vi "main_EMD.vi"() -> ()   [LabVIEW 2018]
uses:
  <vilib>/Utility/file.llb/Read Delimited Spreadsheet (DBL).vi
  <vilib>/express/express analysis/Spectral/Block/exnSpectralBlock spectral measurements PSD poly.vi
  <vilib>/express/express analysis/Spectral/Block/exnSpectralBlock spectral measurements PSD WFM.vi
  <vilib>/express/express analysis/Spectral/XNode/ExpressSpectralMeasurementsBlockNode.xnode
  <vilib>/Analysis/NI_AALPro.lvlib
panel:
  out "PN50":dbl
  out "String":string
  out "LF/HF":dbl
  out "LF":dbl
  out "HF":dbl
  out "integral of P(x)":dbl
  out "Waveform Graph 3":cluster{"f0":dbl, "df":dbl, "magnitude":dbl[]}(graph)
  out "std(ms)":dbl[](array[numeric])
  out "R-R interval(ms)":dbl[](array[numeric])
  out "R wave time":dbl[](array[numeric])
  out "Heart Rate":dbl
  out "Waveform Graph 2":waveform(dbl)(graph)
  out "Ninth_IMF":dbl[](graph)
  out "Waveform Graph":dbl[][](graph)
  out "Eighth IMF":dbl[](graph)
  out "Seventh IMF":dbl[](graph)
  out "Sixth IMF":dbl[](graph)
  out "Fifth IMF":dbl[](graph)
  out "Num of IMF":i32
  out "original signal":dbl[](graph)
  in  "file path (dialog if empty)":path
  out "Fourth IMF":dbl[](graph)
  out "Third IMF":dbl[](graph)
  out "Second IMF":dbl[](graph)
  out "First IMF":dbl[](graph)
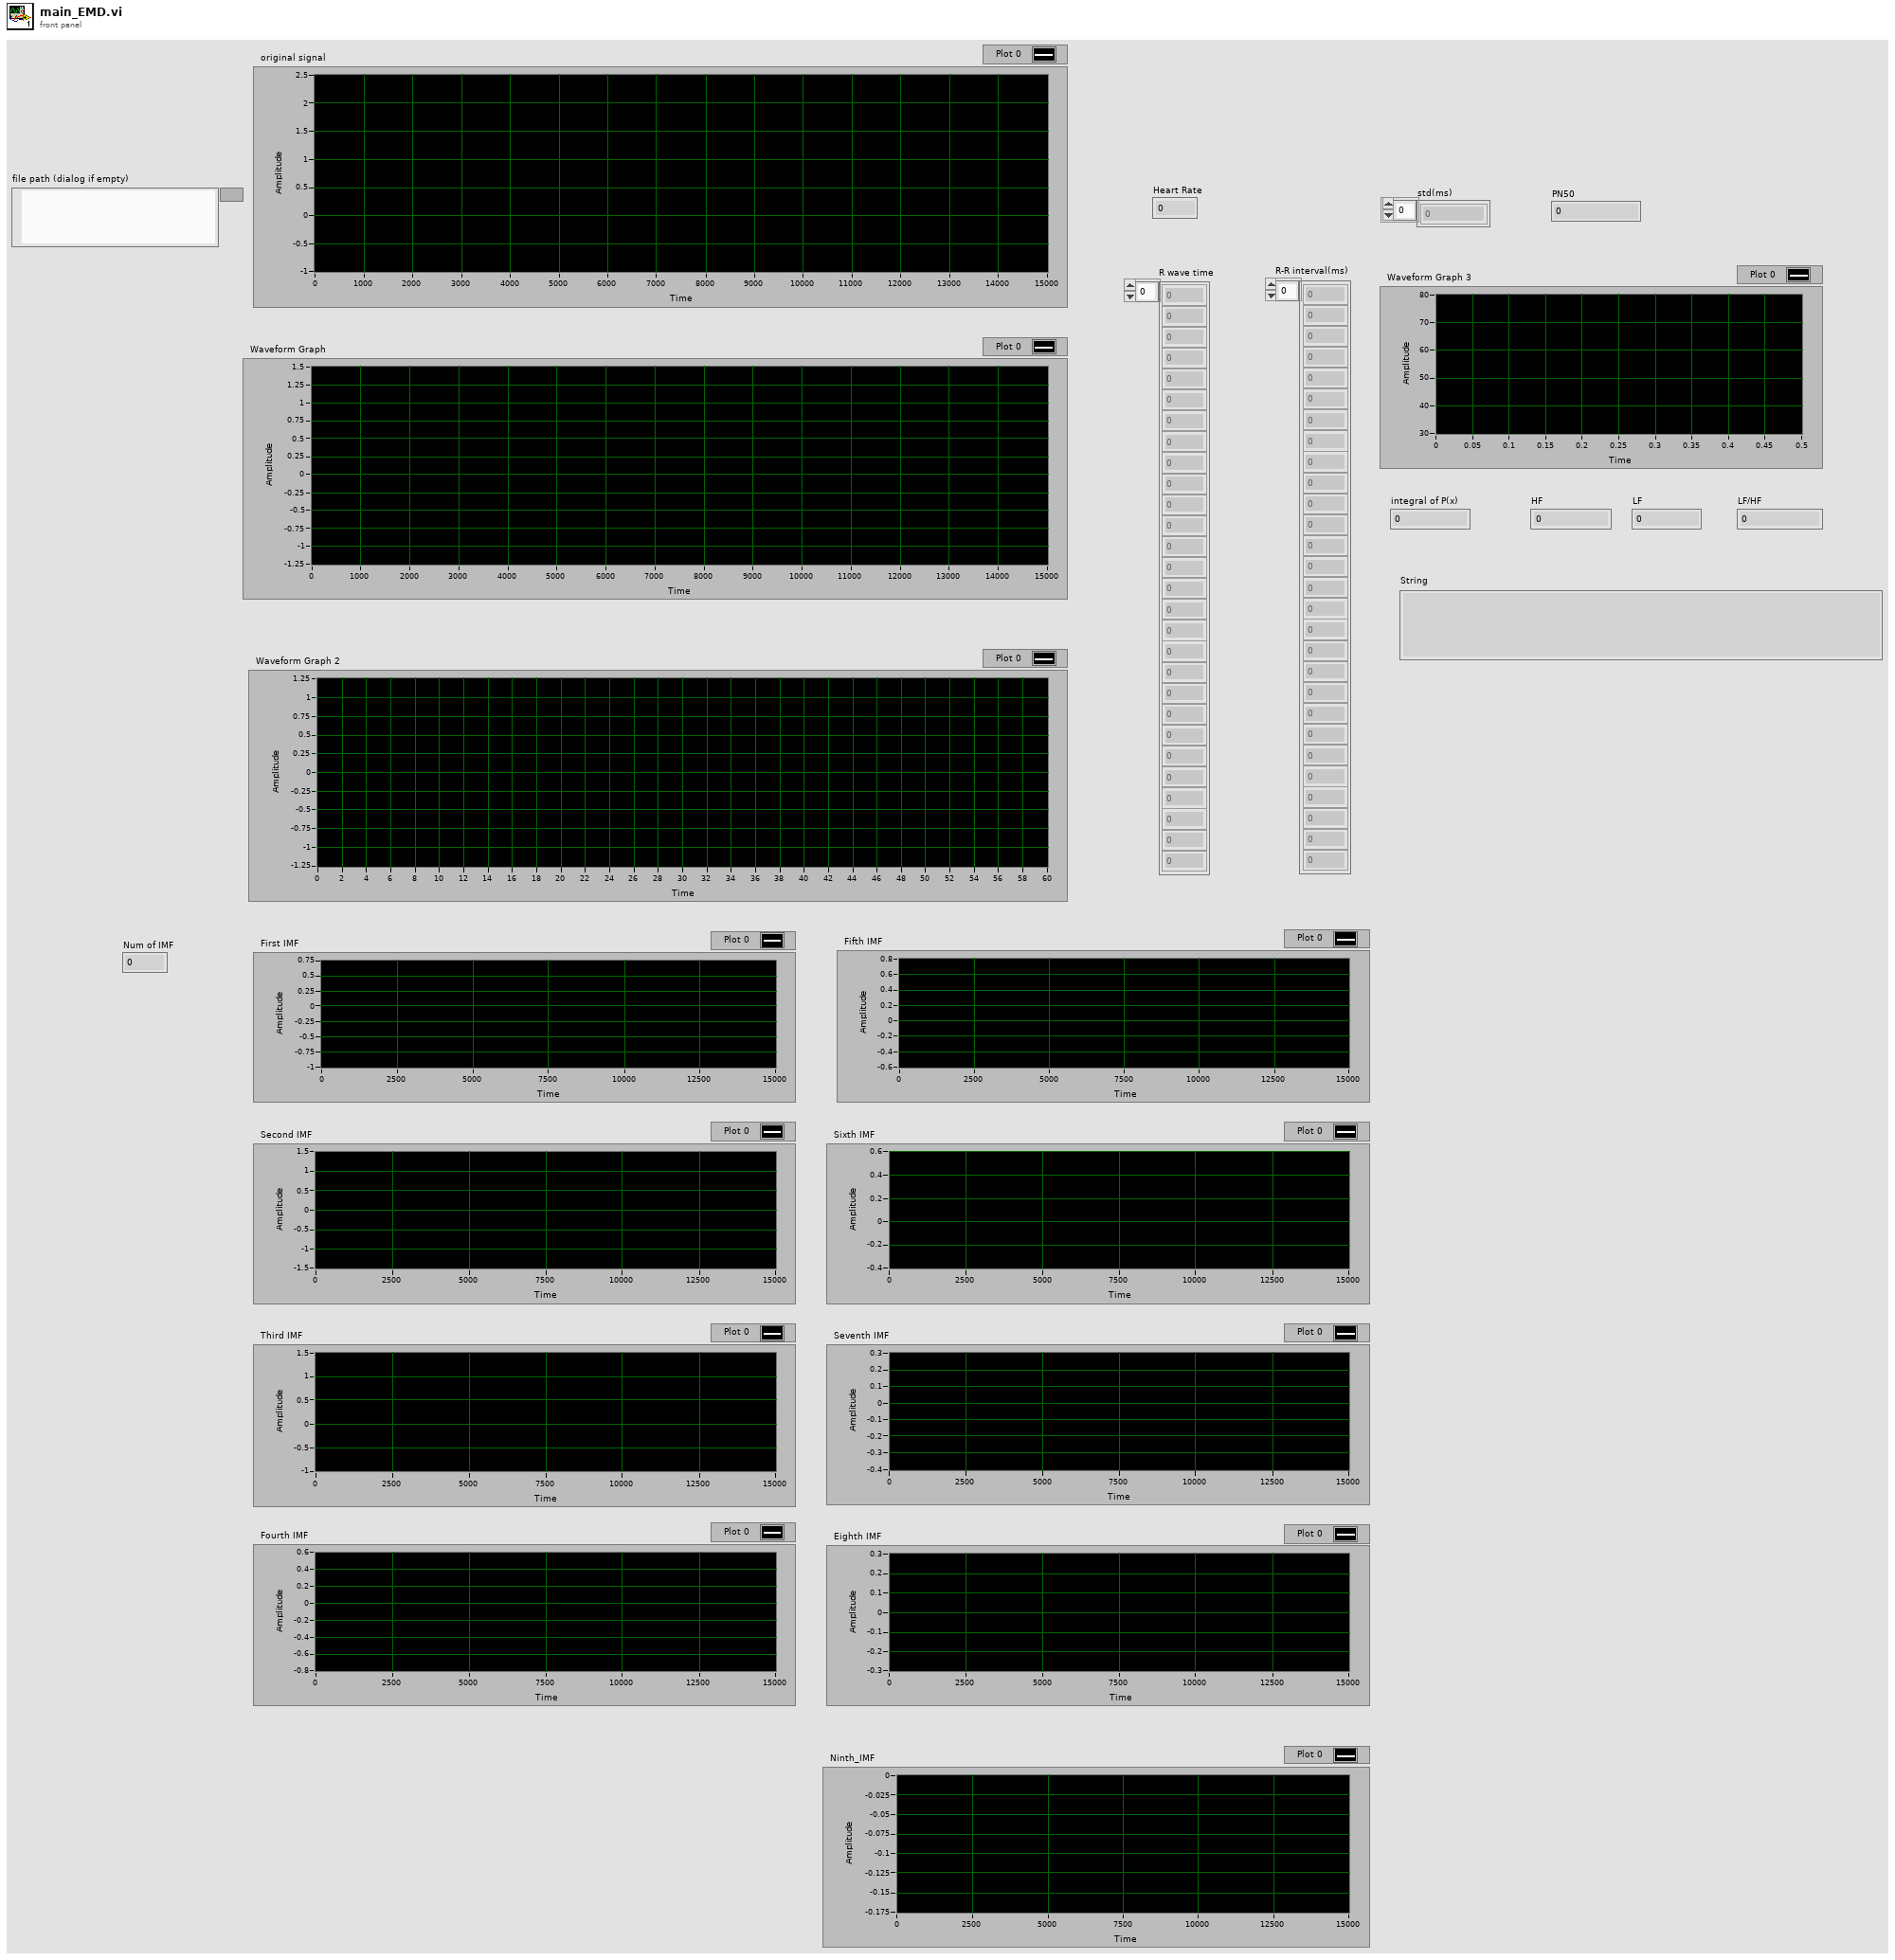
[diagram p1: front panel]
types:
  T1 = cluster{"averaging mode":u16, "weighting mode":u16, "number of averages":u32}
  T2 = cluster{"dB On (F)":bool, "unwrap phase (F)":bool, "convert to degree (F)":bool}
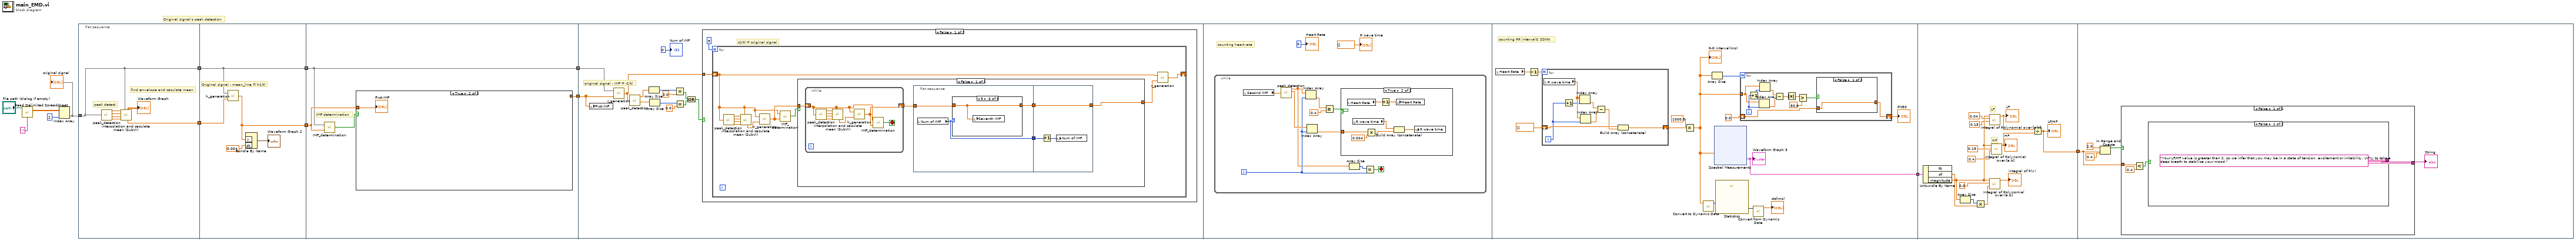
[diagram p0: block diagram]
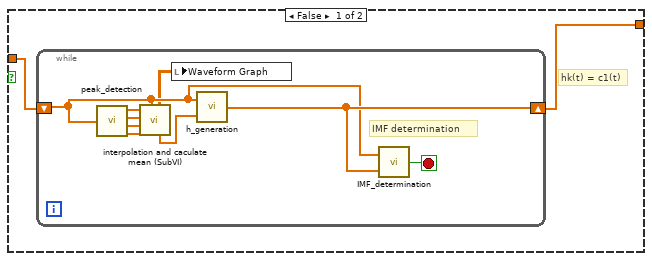
[diagram p2: hidden frame]
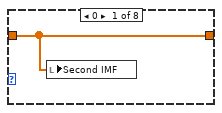
[diagram p3: hidden frame]
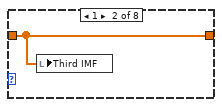
[diagram p4: hidden frame]
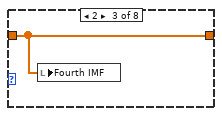
[diagram p5: hidden frame]
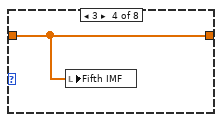
[diagram p6: hidden frame]
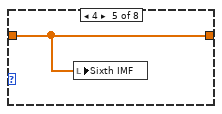
[diagram p7: hidden frame]
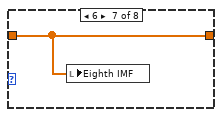
[diagram p8: hidden frame]
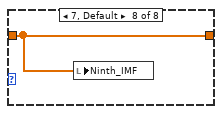
[diagram p9: hidden frame]
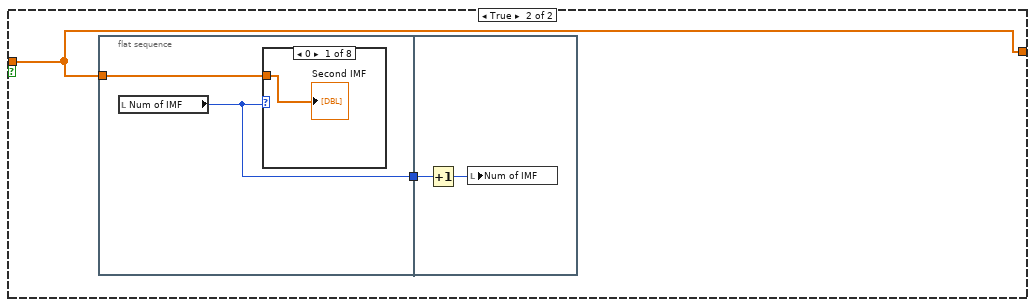
[diagram p10: hidden frame]
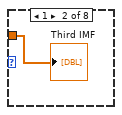
[diagram p11: hidden frame]
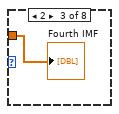
[diagram p12: hidden frame]
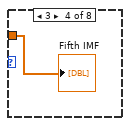
[diagram p13: hidden frame]
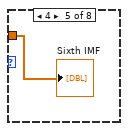
[diagram p14: hidden frame]
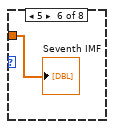
[diagram p15: hidden frame]
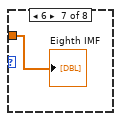
[diagram p16: hidden frame]
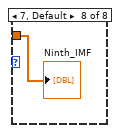
[diagram p17: hidden frame]
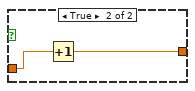
[diagram p20: hidden frame]
diagram:
  # "Original signal's peak detection"
  n1 = call-poly <vilib>:"Read Delimited Spreadsheet.vi"("file path (dialog if empty)"="file path (dialog if empty)", "delimiter (\\t)"=",") -> ("all rows"=w3:dbl[][])  [unwired: 8 in, 5 out]
  n2 = Index Array(array=w3, index (col)=2) -> (element=w4:dbl[])  [unwired: 1 in]
  "original signal" <- w4
  n3 = flat-sequence {
    tunnel: w4 -> [w20]
    tunnel: [w20] -> w13
    tunnel: [w15] -> w9
    tunnel: w13 -> [w25]
    tunnel: [w23] -> w12
    tunnel: [w25] -> w11
    tunnel: w9 -> [w24]
    tunnel: w12 -> [w28]
    tunnel: [w26] -> w8
    tunnel: w11 -> [w26]
    tunnel: [w29] -> w7
    tunnel: w8 -> [w44]
    tunnel: w7 -> [w43]
    tunnel: [w131] -> w2
    tunnel: w2 -> [w184]
    tunnel: [w171] -> w1
    tunnel: w1 -> [w185]
    frame #0 {
      # "peak detect"
      # "find envelope and caculate mean"
      n4 = call "peak_detection.vi"("Array"=w20) -> ("upper"=w19:dbl[], "upper time"=w18:dbl[], "lower"=w17:dbl[], "lower time"=w16:dbl[])
      n5 = call "interpolation and caculate mean (SubVI).vi"("upper"=w19, "upper time"=w18, "lower"=w17, "lower time"=w16, "original"=w20) -> ("up+mean+low"=→"Waveform Graph":dbl[][], "mean after interpolation"=w15:dbl[])  [unwired: 4 out]
    }
    frame #1 {
      # "Original signal - mean_line = h1(t)"
      n6 = call "h_generation.vi"("every_mean_points"=w24, "Y"=w25) -> ("h(t)"=w23:dbl[])
      n7 = Bundle By Name("Y"=w23, "dt"=0.004) -> (→"Waveform Graph 2":waveform(dbl))  [unwired: 1 in]
    }
    frame #2 {
      # "IMF determination"
      n8 = call "IMF_determination.vi"("h(t)"=w28, "original signal"=w26) -> ("x .and. y?"=w27:bool)
      n9 = case shown="True" w27 {
        tunnel: w28 -> [w31 w41]
        tunnel: [w30 _] -> w29
        frame False {
          # "hk(t) = c1(t)"
          n10 = while {
            shift-right: [w35] -> w30
            shift-left: w31 -> [w33]
            stop <- w34 stop-if-true
            # "IMF determination"
            n11 = call "peak_detection.vi"("Array"=w33) -> ("upper"=w40:dbl[], "upper time"=w39:dbl[], "lower"=w38:dbl[], "lower time"=w37:dbl[])
            n12 = call "interpolation and caculate mean (SubVI).vi"("upper"=w40, "upper time"=w39, "lower"=w38, "lower time"=w37, "original"=w33) -> ("up+mean+low"=w32:dbl[][], "mean after interpolation"=w36:dbl[])  [unwired: 4 out]
            n13 = local write "Waveform Graph"(w32) -> ()
            n14 = call "h_generation.vi"("every_mean_points"=w36, "Y"=w33) -> ("h(t)"=w35:dbl[])
            n15 = call "IMF_determination.vi"("h(t)"=w35, "original signal"=w33) -> ("x .and. y?"=w34:bool)
          }
        }
        frame True {
          "First IMF" <- w41
        }
      }
    }
    frame #3 {
      # "original signal - IMF = r1(t)"
      n16 = local write "First IMF"(w43) -> ()
      n17 = call "r_generation.vi"("IMF_points"=w43, "Original_signal"=w44) -> ("r1(t)"=w49:dbl[])
      n18 = call "peak_detection.vi"("Array"=w49) -> ("upper"=w48:dbl[], "lower"=w46:dbl[])  [unwired: 2 out]
      n19 = Array Size(array=w48) -> (size(s)=w47:i32)
      n20 = Array Size(array=w46) -> (size(s)=w45:i32)
      n21 = Equal?(x=w47, y=0.0) -> (x = y?=w52:bool)
      n22 = Equal?(x=w45, y=0.0) -> (x = y?=w51:bool)
      n23 = Or(x=w52, y=w51) -> (x .or. y?=w50:bool)
      n24 = case shown="False" w50 {
        tunnel: w49 -> [w56 _]
        frame False {
          # "c1(t) = original signal"
          n25 = for {
            N: 9 -> [_]
            shift-right: [w57] -> _
            shift-left: w56 -> [w59]
            n26 = call "peak_detection.vi"("Array"=w59) -> ("upper"=w66:dbl[], "upper time"=w65:dbl[], "lower"=w64:dbl[], "lower time"=w63:dbl[])
            n27 = call "interpolation and caculate mean (SubVI).vi"("upper"=w66, "upper time"=w65, "lower"=w64, "lower time"=w63, "original"=w59) -> ("mean after interpolation"=w62:dbl[])  [unwired: 5 out]
            n28 = call "h_generation.vi"("every_mean_points"=w62, "Y"=w59) -> ("h(t)"=w61:dbl[])
            n29 = call "IMF_determination.vi"("h(t)"=w61, "original signal"=w59) -> ("x .and. y?"=w60:bool)
            n30 = case shown="False" w60 {
              tunnel: w61 -> [w71 w94]
              tunnel: [w69 w94] -> w58
              frame False {
                n31 = while {
                  shift-right: [w87] -> w70
                  shift-left: w71 -> [w86]
                  stop <- w88 stop-if-true
                  n32 = call "peak_detection.vi"("Array"=w86) -> ("upper"=w93:dbl[], "upper time"=w92:dbl[], "lower"=w91:dbl[], "lower time"=w90:dbl[])
                  n33 = call "interpolation and caculate mean (SubVI).vi"("upper"=w93, "upper time"=w92, "lower"=w91, "lower time"=w90, "original"=w86) -> ("mean after interpolation"=w89:dbl[])  [unwired: 5 out]
                  n34 = call "h_generation.vi"("every_mean_points"=w89, "Y"=w86) -> ("h(t)"=w87:dbl[])
                  n35 = call "IMF_determination.vi"("h(t)"=w87, "original signal"=w86) -> ("x .and. y?"=w88:bool)
                }
                n36 = flat-sequence {
                  tunnel: w70 -> [w74]
                  tunnel: [w73] -> w68
                  tunnel: [w72] -> w67
                  tunnel: [w85] -> w69
                  tunnel: w68 -> [w85]
                  tunnel: w67 -> [w84]
                  frame #0 {
                    n37 = local read "Num of IMF"() -> (w72:i32)
                    n38 = case shown="5" w72 {
                      tunnel: w74 -> [w75 w76 w77 w78 w79 w80 w81 w82]
                      tunnel: [w75 w76 w77 w78 w79 w80 w81 w82] -> w73
                      frame 0 {
                        n39 = local write "Second IMF"(w75) -> ()
                      }
                      frame 1 {
                        n40 = local write "Third IMF"(w76) -> ()
                      }
                      frame 2 {
                        n41 = local write "Fourth IMF"(w77) -> ()
                      }
                      frame 3 {
                        n42 = local write "Fifth IMF"(w78) -> ()
                      }
                      frame 4 {
                        n43 = local write "Sixth IMF"(w79) -> ()
                      }
                      frame 5 {
                        n44 = local write "Seventh IMF"(w80) -> ()
                      }
                      frame 6 {
                        n45 = local write "Eighth IMF"(w81) -> ()
                      }
                      frame 7, Default {
                        n46 = local write "Ninth_IMF"(w82) -> ()
                      }
                    }
                  }
                  frame #1 {
                    n47 = Increment(x=w84) -> (x+1=w83:i32)
                    n48 = local write "Num of IMF"(w83) -> ()
                  }
                }
              }
              frame True {
                n49 = flat-sequence {
                  tunnel: w94 -> [w97]
                  tunnel: [w96] -> w95
                  tunnel: w95 -> [w107]
                  frame #0 {
                    n50 = local read "Num of IMF"() -> (w96:i32)
                    n51 = case shown="0" w96 {
                      tunnel: w97 -> [w98 w99 w100 w101 w102 w103 w104 w105]
                      frame 0 {
                        "Second IMF" <- w98
                      }
                      frame 1 {
                        "Third IMF" <- w99
                      }
                      frame 2 {
                        "Fourth IMF" <- w100
                      }
                      frame 3 {
                        "Fifth IMF" <- w101
                      }
                      frame 4 {
                        "Sixth IMF" <- w102
                      }
                      frame 5 {
                        "Seventh IMF" <- w103
                      }
                      frame 6 {
                        "Eighth IMF" <- w104
                      }
                      frame 7, Default {
                        "Ninth_IMF" <- w105
                      }
                    }
                  }
                  frame #1 {
                    n52 = Increment(x=w107) -> (x+1=w106:i32)
                    n53 = local write "Num of IMF"(w106) -> ()
                  }
                }
              }
            }
            n54 = call "r_generation.vi"("IMF_points"=w58, "Original_signal"=w59) -> ("r1(t)"=w57:dbl[])
          }
        }
        frame True {
        }
      }
      "Num of IMF" <- 0
    }
    frame #4 {
      # "counting heart rate"
      n55 = while {
        i -> [w113]
        stop <- w118 stop-if-true
        n56 = local read "Second IMF"() -> (w110:dbl[])
        n57 = call "peak_detection.vi"("Array"=w110) -> ("upper"=w111:dbl[], "upper time"=w114:dbl[])  [unwired: 2 out]
        n58 = Index Array(array=w111, index=w113) -> (element=w117:dbl)
        n59 = Index Array(array=w114, index=w113) -> (element=w112:dbl)
        n60 = Greater Or Equal?(x=w117, y=0.4) -> (x >= y?=w115:bool)
        n61 = case shown="True" w115 {
          tunnel: w112 -> [_ w124]
          frame False {
          }
          frame True {
            n62 = local read "Heart Rate"() -> (w125:dbl)
            n63 = local read "R wave time"() -> (w121:dbl[])
            n64 = Multiply(x=w124, y=0.004) -> (x*y=w122:dbl)
            n65 = Increment(x=w125) -> (x+1=w126:dbl)
            n66 = Build Array (concatenate)(w121, w122) -> (w120:dbl[])
            n67 = local write "Heart Rate"(w126) -> ()
            n68 = local write "R wave time"(w120) -> ()
          }
        }
        n69 = Array Size(array=w111) -> (size(s)=w119:i32)
        n70 = Equal?(x=w119, y=w113) -> (x = y?=w118:bool)
      }
      "Heart Rate" <- 0
      "R wave time" <- dbl[] []
    }
    frame #5 {
      # "counting RR interval& SDNN"
      n71 = local read "Heart Rate"() -> (w138:dbl)
      n72 = Decrement(x=w138) -> (x-1=w137:dbl)
      n73 = for {
        N: w137 -> [_]
        shift-right: [w163] -> w133
        shift-left: dbl[] [] -> [w164]
        i -> [w166]
        n74 = local read "R wave time"() -> (w170:dbl[])
        n75 = Increment(x=w166) -> (x+1=w169:i32)
        n76 = Index Array(array=w170, index=w169) -> (element=w168:dbl)
        n77 = Index Array(array=w170, index=w166) -> (element=w167:dbl)
        n78 = Subtract(x=w168, y=w167) -> (x-y=w165:dbl)
        n79 = Build Array (concatenate)(w164, w165) -> (w163:dbl[])
      }
      n80 = Multiply(x=1000.0, y=w133) -> (x*y=w129:dbl[])
      "R-R interval(ms)" <- w129
      n81 = call "Convert to Dynamic Data"("Array"=w129) -> ("Dynamic Data Type"=w136:dynamicdata)  [unwired: 3 in]
      n82 = Array Size(array=w129) -> (size(s)=w130:i32)
      n83 = xnode "Spectral Measurements"("Signals"=w129) -> ("PSD"=w131:cluster{"f0":dbl, "df":dbl, "magnitude":dbl[]})  [unwired: 1 in, 1 out]
      "Waveform Graph 3" <- w131
      n84 = call "Statistics"("Signals"=w136) -> ("Standard Dev"=w135:dynamicdata)  [unwired: 25 in, 1 out]
      n85 = for {
        N: w130 -> [_]
        tunnel: w129 -> [w148]
        shift-right: [w140] -> w128
        shift-left: 0.0 -> [w141]
        i -> [w149]
        n86 = Increment(x=w149) -> (x+1=w150:i32)
        n87 = Index Array(array=w148, index=w149) -> (element=w147:dbl)
        n88 = Index Array(array=w148, index=w150) -> (element=w146:dbl)
        n89 = Subtract(x=w146, y=w147) -> (x-y=w145:dbl)
        n90 = Absolute Value(x=w145) -> (abs(x)=w144:dbl)
        n91 = Greater?(x=w144, y=50.0) -> (0:w142:bool)
        n92 = case shown="False" w142 {
          tunnel: w141 -> [w151 w153]
          tunnel: [w151 w152] -> w140
          frame False {
          }
          frame True {
            n93 = Increment(x=w153) -> (x+1=w152:dbl)
          }
        }
      }
      "PN50" <- w128
      n94 = call "Convert from Dynamic Data"("Dynamic Data Type"=w135) -> ("Array"=→"std(ms)":dbl[])  [unwired: 3 in]
    }
    frame #6 {
      # "LF"
      # "HF"
      n95 = Unbundle By Name(w184) -> ("df"=w179:dbl, "magnitude"=w176:dbl[])  [unwired: 1 out]
      n96 = Array Size(array=w176) -> (size(s)=w182:i32)
      n97 = Multiply(x=w182, y=w179) -> (x*y=w181:dbl)
      n98 = call <vilib>:"Integral of Polynomial over [a,b].vi"("b"=0.15, "a"=0.04, "P(x)"=w176) -> ("integral of P(x)"=w173:dbl)  [unwired: 7 in, 1 out]
      "LF" <- w173
      n99 = call <vilib>:"Integral of Polynomial over [a,b].vi"("b"=w181, "a"=0.0, "P(x)"=w176) -> ("integral of P(x)"=→"integral of P(x)":dbl)  [unwired: 7 in, 1 out]
      n100 = call <vilib>:"Integral of Polynomial over [a,b].vi"("b"=0.4, "a"=0.15, "P(x)"=w176) -> ("integral of P(x)"=w172:dbl)  [unwired: 7 in, 1 out]
      "HF" <- w172
      n101 = Divide(x=w173, y=w172) -> (x/y=w171:dbl)
      "LF/HF" <- w171
    }
    frame #7 {
      n102 = In Range and Coerce(upper limit=2.0, x=w185, lower limit=0.4) -> (In Range?=w187:bool)  [unwired: 1 out]
      n103 = case shown="False" w187 {
        tunnel: [w190 "Your LF/HL value is within the normal range. \nWe assume that your mood is comfortable and stable. \nPlease keep it up."] -> w186
        tunnel: w185 -> [w191 _]
        frame False {
          n104 = Less?(x=w191, y=0.4) -> (x < y?=w193:bool)
          n105 = case shown="False" w193 {
            tunnel: ["Your LF/HF value is greater than 2, so we infer that you may be in a state of tension, excitement or irritability. \nTry to take a deep breath to stabilize your mood." "Your LF/HF value is less than 0.4, so we speculate that you are in a state of depression.\nI suggest you go out for a walk to watch the scenery or chat with friends."] -> w190
            frame False {
            }
            frame True {
            }
          }
        }
        frame True {
        }
      }
      "String" <- w186
    }
  }
